vi "AutoCAD cmds 64bit.vi"(6 "AutoCAD cmd":T3, 8 "error in (no error)":errorcluster, 9 "Command":string, 10 "Mathcad Output":T2, 11 "DesignRequest":T1) -> (0 "error out":errorcluster, 2 "IsQuiescent":bool, 3 "DesignRequest out":T1)   [LabVIEW 2011, in "Design Server.lvlib"]
uses:
  Design Server.lvlib
  AutoCAD cmds.ctl
  Variable cluster.ctl
  Design Request.ctl
panel:
  in  "Path":path=path "C:/Users/design/AppData/Local/Autodesk/AutoCAD 2012 - English/R18.2/enu/Template/AguaClara.dwt"
  out "wating":i32
  out "new doc error":errorcluster
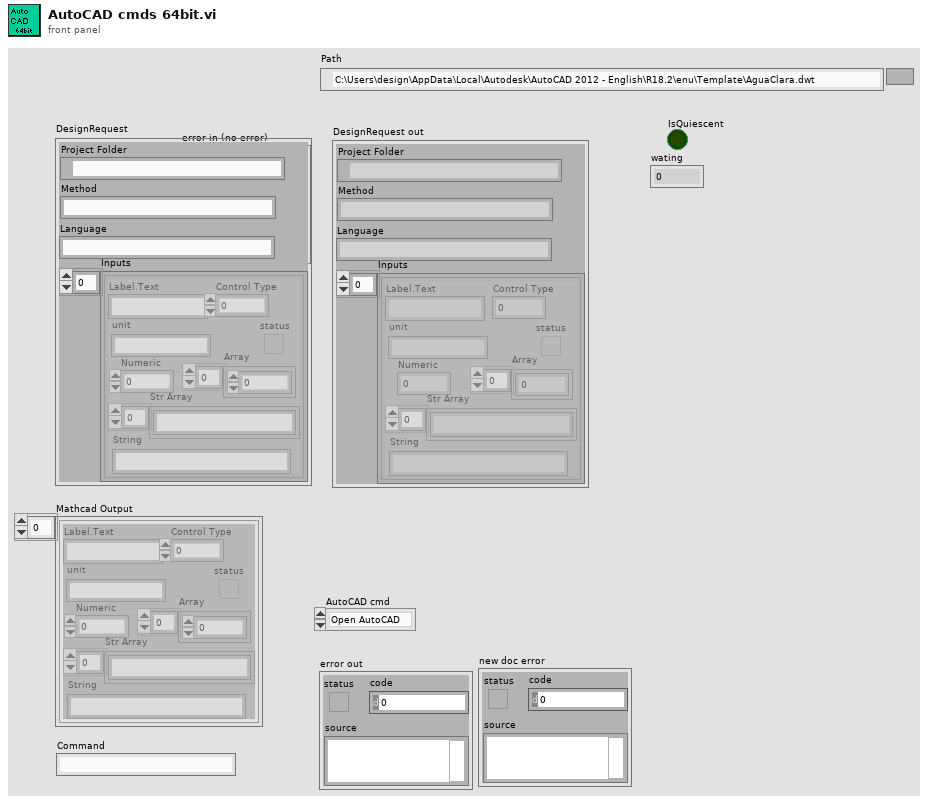
[diagram p1: front panel]
types:
  T1 = typedef "Design Server.lvlib/Design Request.ctl" = cluster{"Project Folder":path, "Method":string, "Inputs":T2, "Language":string}
  T2 = typedef "Design Server.lvlib/Variable cluster.ctl" = cluster{"Label.Text":string, "Control Type":u32, "Numeric":dbl, "Array":dbl[], "status":bool, "Str Array":string[], "String":string, "unit":string}[]
  T3 = typedef "Design Server.lvlib/AutoCAD cmds.ctl" = enum16{"Open AutoCAD", "Create Drawing", "Quit"}
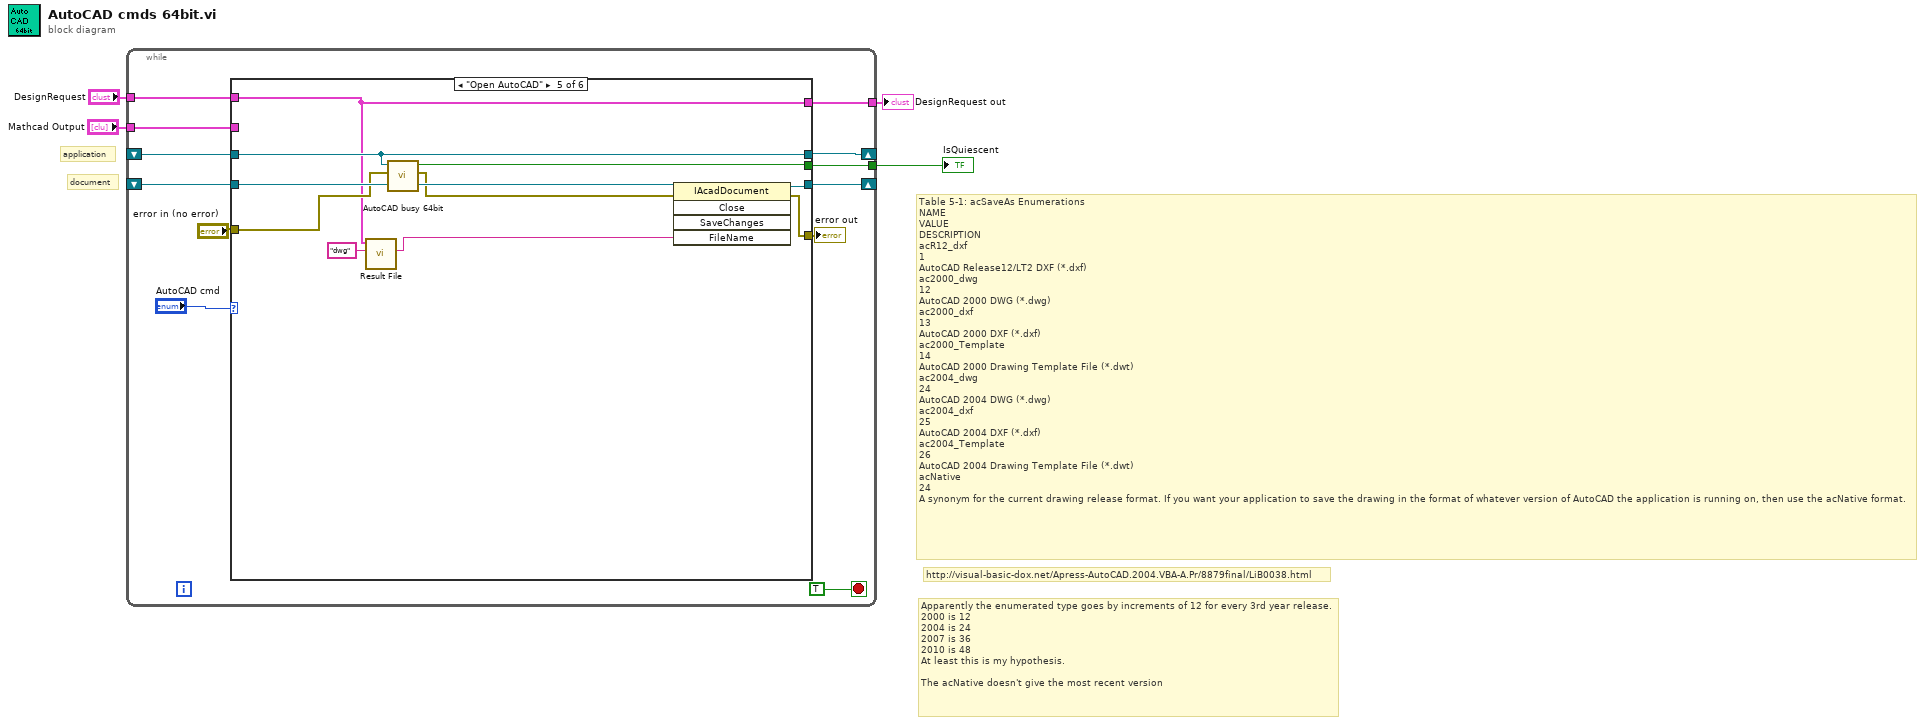
[diagram p0: block diagram]
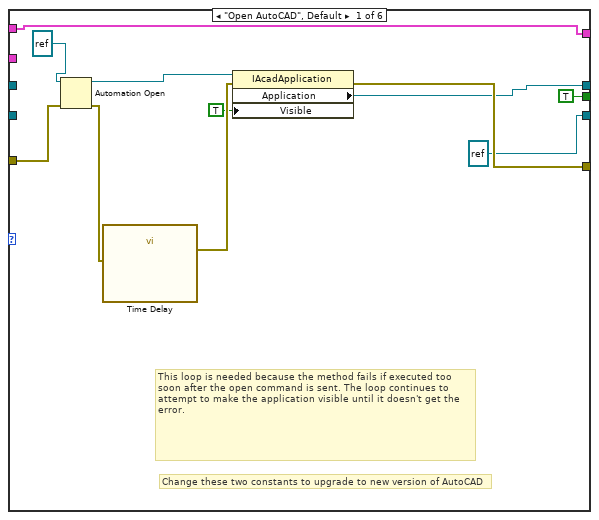
[diagram p2: hidden frame]
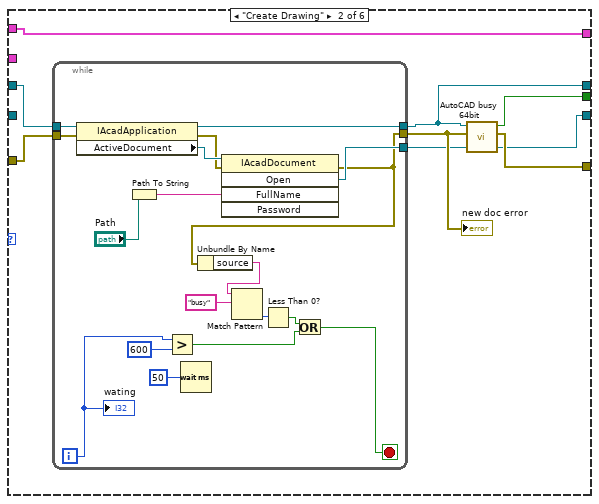
[diagram p3: hidden frame]
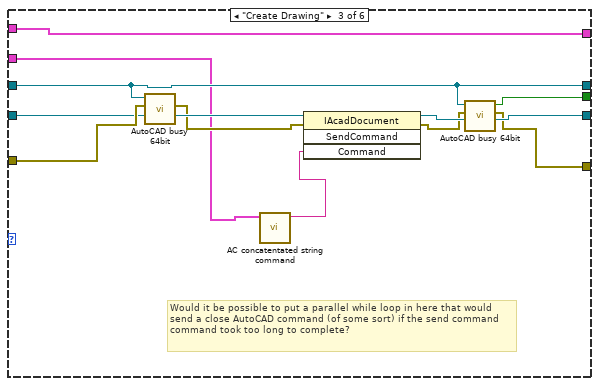
[diagram p4: hidden frame]
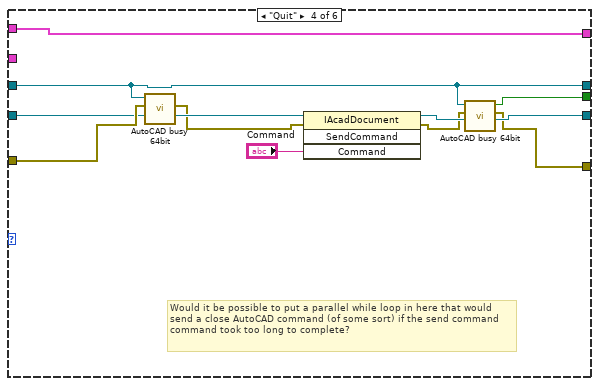
[diagram p5: hidden frame]
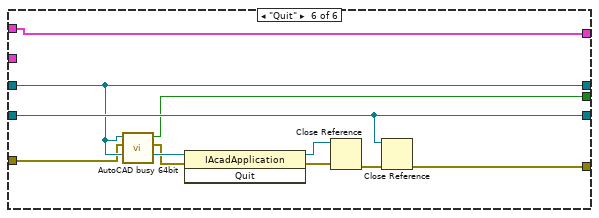
[diagram p6: hidden frame]
diagram:
  # "Apparently the enumerated type goes by increments of 12 for every 3rd year release.\n2000 is 12\n2004 is 24\n2007 is 36\n2010 is 48\nAt least this is my hypothesis. \n\nThe acNative doesn't give the most recent version"
  # "http://visual-basic-dox.net/Apress-AutoCAD.2004.VBA-A.Pr/8879final/LiB0038.html"
  # "Table 5-1: acSaveAs Enumerations\nNAME\nVALUE\nDESCRIPTION\nacR12_dxf\n1\nAutoCAD Release12/LT2 DXF (*.dxf)\nac2000_dwg\n12\nAutoCAD 2000 DWG (*.dwg)\nac2000_dxf\n13\nAutoCAD 2000 DXF (*.dxf)\nac2000_Template\n14\nAutoCAD 2000 Drawing Template File (*.dwt)\nac2004_dwg\n24\nAutoCAD 2004 DWG (*.dwg)\nac2004_dxf\n25\nAutoCAD 2004 DXF (*.dxf)\nac2004_Template\n26\nAutoCAD 2004 Drawing Template File (*.dwt)\nacNative\n24\nA synonym for the current drawing release format. If you want your application to save the drawing in the format of whatever version of AutoCAD the application is running on, then use the acNative format."
  # "document"
  # "application"
  n1 = while {
    shift-right: [w15] -> _
    shift-left: _ -> [w10]
    shift-right: [w12] -> _
    shift-left: _ -> [w11]
    tunnel: [w8] -> w4
    tunnel: [w7] -> w3
    tunnel: "DesignRequest" -> [w6]
    tunnel: "Mathcad Output" -> [w5]
    stop <- TRUE stop-if-true
    n2 = case shown="\"Close Doc\"" "AutoCAD cmd" {
      tunnel: [w24 w28 w59 w70 w81 w89] -> w15
      tunnel: "error in (no error)" -> [w21 w29 w64 w74 w80 w88]
      tunnel: [w27 w35 w57 w68 w82 w90] -> w13
      tunnel: [refnum<k7> refnum ("Add") w31 w61 w71 w83 w91] -> w12
      tunnel: w11 -> [_ _ w63 w73 w84 w91]
      tunnel: w10 -> [_ w33 w59 w70 w81 w89]
      tunnel: [TRUE ("IsQuiescent") w34 w56 w67 w78 w86] -> w8
      tunnel: [w18 w30 w54 w66 w75 w85] -> w7
      tunnel: w6 -> [w18 w30 w54 w66 w75 w85]
      tunnel: w5 -> [_ _ w55 _ _ _]
      frame "Open AutoCAD", Default {
        # "This loop is needed because the method fails if executed too soon after the open command is sent. The loop continues to attempt to make the application visible until it doesn't get the error."
        # "Change these two constants to upgrade to new version of AutoCAD"
        n3 = Automation Open(error in (no error)=w21, Automation Refnum=refnum<k7> refnum ("reference")) -> (Automation Refnum=w22:refnum<k7>, error out=w20:errorcluster)  [unwired: 2 in]
        n4 = call "Time Delay"("error in (no error)"=w20) -> ("error out"=w19:errorcluster)  [unwired: 10 in]
        n5 = property class="IAcadApplication"(reference=w22, error in=w19, "Visible"=TRUE) -> (error out=w27:errorcluster, "Application"=w24:refnum<k7>)  [unwired: 1 out]
      }
      frame "Create Drawing" {
        n6 = while {
          tunnel: w33 -> [w45]
          tunnel: [w43] -> w28
          tunnel: [w38] -> w32
          tunnel: [w40] -> w31
          tunnel: w29 -> [w44]
          i -> [w49]
          stop <- w46 stop-if-true
          n7 = property class="IAcadApplication"(reference=w45, error in=w44) -> (reference out=w43:refnum<k7>, error out=w39:errorcluster, "ActiveDocument"=w41:refnum<k7>)
          n8 = Path To String(path="Path") -> (string=w36:string)
          n9 = Greater?(x=w49, y=600) -> (0:w47:bool)
          n10 = Wait (ms)(milliseconds to wait=u32 50) -> ()  [unwired: 1 out]
          n11 = invoke class="IAcadDocument" method="Open"(reference=w41, error in=w39, "FullName"=w36) -> (error out=w38:errorcluster, "Open"=w40:refnum<k7>)  [unwired: 2 in, 3 out]
          n12 = Unbundle By Name(w38) -> ("source"=w42:string)
          n13 = Match Pattern(string=w42, regular expression="busy") -> (offset past match=w52:i32)  [unwired: 1 in, 3 out]
          n14 = Less Than 0?(x=w52) -> (x < 0?=w48:bool)
          n15 = Or(x=w48, y=w47) -> (x .or. y?=w46:bool)
          "wating" <- w49
        }
        "new doc error" <- w32
        n16 = call "AutoCAD busy 64bit.vi"("error in (no error)"=w32, "Application"=w28) -> ("error out"=w35:errorcluster, "IsQuiescent"=w34:bool)  [unwired: 4 in]
      }
      frame "Create Drawing" {
        # "Would it be possible to put a parallel while loop in here that would send a close AutoCAD command (of some sort) if the send command command took too long to complete?"
        n17 = call "AutoCAD busy 64bit.vi"("error in (no error)"=w64, "Application"=w59) -> ("error out"=w62:errorcluster)  [unwired: 4 in, 1 out]
        n18 = call "AC concatentated string command.vi"("MathCAD results"=w55) -> ("AC concatenated string"=w60:string)  [unwired: 10 in]
        n19 = invoke class="IAcadDocument" method="SendCommand"(reference=w63, error in=w62, "Command"=w60) -> (reference out=w61:refnum<k7>, error out=w58:errorcluster)  [unwired: 1 in, 2 out]
        n20 = call "AutoCAD busy 64bit.vi"("error in (no error)"=w58, "Application"=w59) -> ("error out"=w57:errorcluster, "IsQuiescent"=w56:bool)  [unwired: 4 in]
      }
      frame "Quit" {
        # "Would it be possible to put a parallel while loop in here that would send a close AutoCAD command (of some sort) if the send command command took too long to complete?"
        n21 = call "AutoCAD busy 64bit.vi"("error in (no error)"=w74, "Application"=w70) -> ("error out"=w72:errorcluster)  [unwired: 4 in, 1 out]
        n22 = invoke class="IAcadDocument" method="SendCommand"(reference=w73, error in=w72, "Command"="Command") -> (reference out=w71:refnum<k7>, error out=w69:errorcluster)  [unwired: 1 in, 2 out]
        n23 = call "AutoCAD busy 64bit.vi"("error in (no error)"=w69, "Application"=w70) -> ("error out"=w68:errorcluster, "IsQuiescent"=w67:bool)  [unwired: 4 in]
      }
      frame "Open AutoCAD" {
        n24 = call "Result File.vi"("File Type"="dwg", "DesignRequest"=w75) -> ("File string"=w76:string)  [unwired: 8 in, 1 out]
        n25 = call "AutoCAD busy 64bit.vi"("error in (no error)"=w80, "Application"=w81) -> ("error out"=w79:errorcluster, "IsQuiescent"=w78:bool)  [unwired: 4 in]
        n26 = invoke class="IAcadDocument" method="Close"(reference=w84, error in=w79, "FileName"=w76) -> (reference out=w83:refnum<k7>, error out=w82:errorcluster)  [unwired: 2 in, 3 out]
      }
      frame "Quit" {
        n27 = call "AutoCAD busy 64bit.vi"("error in (no error)"=w88, "Application"=w89) -> ("error out"=w87:errorcluster, "IsQuiescent"=w86:bool)  [unwired: 4 in]
        n28 = invoke class="IAcadApplication" method="Quit"(reference=w89, error in=w87) -> (reference out=w94:refnum<k7>, error out=w93:errorcluster)  [unwired: 1 in, 1 out]
        n29 = Close Reference(reference=w94, error in (no error)=w93) -> (error out=w92:errorcluster)
        n30 = Close Reference(reference=w91, error in (no error)=w92) -> (error out=w90:errorcluster)
      }
    }
    "error out" <- w13
  }
  "IsQuiescent" <- w4
  "DesignRequest out" <- w3
